vi "Y[i]=X[i-n] PtByPt.vi"(2 "initialize":bool, 3 "shifts: n":i32, 5 "x":dbl format="%0.2f") -> (0 "error":i32, 1 "shifted x":dbl format="%0.2f")   [LabVIEW 2020, in "NI_PtbyPt.lvlib"]
doc: "Shifts <B>x</B> by <B>shifts: n</B> samples."
uses:
  <vilib>/ptbypt/NI_PtbyPt.lvlib
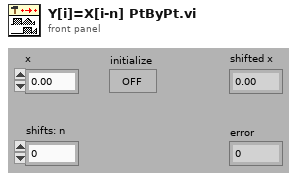
[diagram p1: front panel]
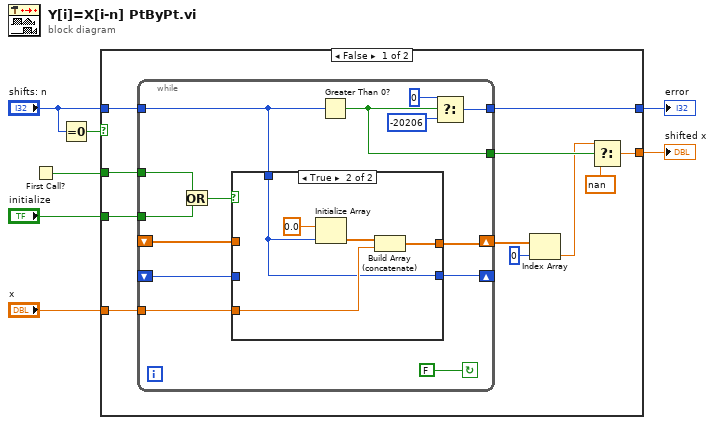
[diagram p0: block diagram]
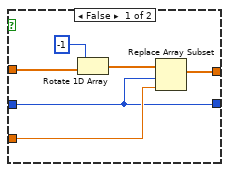
[diagram p2: hidden frame]
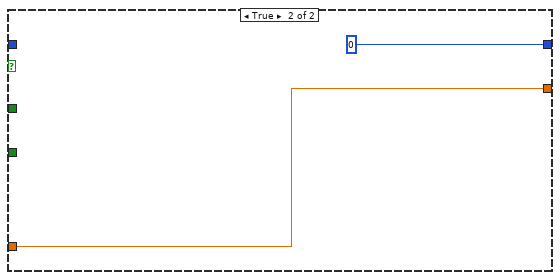
[diagram p3: hidden frame]
diagram:
  n1 = First Call?() -> (First Call?: T/F=w1:bool)
  n2 = Equal To 0?(x="shifts: n") -> (x = 0?=w3:bool)
  n3 = case shown="False" w3 {
    tunnel: "x" -> [w16 w44]
    tunnel: [w8 w44] -> w6
    tunnel: [w14 0 ("error")] -> w5
    tunnel: "shifts: n" -> [w15 _]
    tunnel: "initialize" -> [w18 _]
    tunnel: w1 -> [w17 _]
    frame False {
      n4 = while {
        tunnel: [w20] -> w14
        tunnel: w15 -> [w21]
        tunnel: w16 -> [w24]
        tunnel: w17 -> [w25]
        tunnel: w18 -> [w26]
        shift-left: _ -> [w30]
        shift-right: [w31] -> _
        shift-left: _ -> [w29]
        shift-right: [w32] -> w12
        tunnel: [w19] -> w11
        stop <- FALSE continue-if-true
        n5 = Or(x=w25, y=w26) -> (x .or. y?=w27:bool)
        n6 = case shown="True" w27 {
          tunnel: [w36 w42] -> w32
          tunnel: [w33 w40] -> w31
          tunnel: w30 -> [w33 _]
          tunnel: w29 -> [w34 _]
          tunnel: w24 -> [w37 w43]
          tunnel: w21 -> [_ w40]
          frame False {
            n7 = Rotate 1D Array(1:w34, 2:i16 -1 ("n")) -> (0:w35:dbl[])
            n8 = Replace Array Subset(array=w35, new element=w37, index=w33) -> (w36:dbl[])
          }
          frame True {
            n9 = Initialize Array(0.0, w40) -> (w41:dbl[])
            n10 = Build Array (concatenate)(w41, w43) -> (w42:dbl[])
          }
        }
        n11 = Greater Than 0?(x=w21) -> (x > 0?=w19:bool)
        n12 = Select(t=0, s=w19, f=-20206) -> (s? t:f=w20:i32)
      }
      n13 = Index Array(array=w12, index=0 ("Index")) -> (element=w10:dbl)
      n14 = Select(t=w10, s=w11, f=nan) -> (s? t:f=w8:dbl)
    }
    frame True {
    }
  }
  "shifted x" <- w6
  "error" <- w5
